vi "系列号查询.vi"() -> ()   [LabVIEW 2016, in "斯坦道多参数.lvlib"]
panel:
  in  "传感器系列号":T1
  in  "布尔":bool
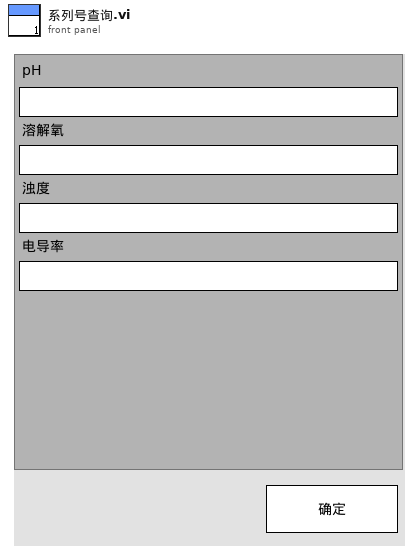
[diagram p1: front panel]
types:
  T1 = cluster{"pH":string, "溶解氧":string, "浊度":string, "电导率":string, "ORP":string, "叶绿素a":string, "藻密度":string}
  T2 = cluster{"pH探头选择":u16, "DO探头选择":u16, "电导率探头选择":u16, "浊度探头选择":u16, "叶绿素a探头选择":u16, "蓝绿藻探头选择":u16, "orp探头选择":u16, "COD探头选择":u16, "DO2探头选择":u16}
  T3 = cluster{"电极状态标志":u16, "电极型号标志":u16, "酸碱度测量值":sgl, "温度测量值":sgl, "酸碱度信号值":sgl, "温度信号值":sgl, "酸碱度偏移修正值":sgl, "温度偏移修正值":sgl, "手动温度补偿值":sgl, "酸碱度电极零点":sgl, "酸碱度电极斜率":sgl, "第1点标准值记录":sgl, "第1点信号值记录":sgl, "第1点温度值记录":sgl, "第2点标准值记录":sgl, "第2点信号值记录":sgl, "第2点温度值记录":sgl, "命令滤波设定":u16, "温度模式":enum16{"ATC", "MTC"}, "生产批次":u16, "电极序号":u16, "串口地址":u16, "串口波特率":enum16{"9600", "19200", "115200"}, "串口校验位":enum16{"NONE", "ODD", "EVEN"}, "串口停止位":enum16{"1bit", "2bit"}, "第一点标准值":sgl, "第二点标准值":sgl}
  T4 = cluster{"报警码":u16, "pH数值":sgl, "0X0003_NC":sgl, "温度数据":sgl, "pH原始信号 mv":sgl, "0X0009_NC":string, "产品名称":string, "序列号":string, "硬件版本":string, "软件版本":string, "通讯地址":u16, "波特率":u16, "设备类型":u16, "0X0026_NC":string, "第一点原始数据":sgl, "第一点校准数据":sgl, "第二点原始数据":sgl, "第二点校准数据":sgl, "探头校准命令":u16, "温度校准参数":sgl, "温度校准命令":u16}
  T5 = cluster{"电极状态标志":u16, "电极型号标志":u16, "溶解氧测量值":sgl, "温度测量值":sgl, "溶解氧饱和度值":sgl, "盐度补偿值":sgl, "大气压补偿值":sgl, "溶解氧偏移修正值":sgl, "温度偏移修正值":sgl, "手动温度补偿值":sgl, "溶解氧电极零点":sgl, "溶解氧电极斜率":sgl, "第1点标准值记录":sgl, "第1点信号值记录":sgl, "第1点温度值记录":sgl, "第2点标准值记录":sgl, "第2点信号值记录":sgl, "第2点温度值记录":sgl, "命令滤波设定":u16, "温度模式":enum16{"ATC", "MTC"}, "生产批次":u16, "电极序号":u16, "串口地址":u16, "串口波特率":enum16{"9600", "19200", "115200"}, "串口校验位":enum16{"NONE", "ODD", "EVEN"}, "串口停止位":enum16{"1bit", "2bit"}, "第一点标准值":sgl, "第二点标准值":sgl}
  T6 = cluster{"报警码":u16, "溶解氧数值（mg/L）":sgl, "溶解氧数据（%）":sgl, "温度数据":sgl, "溶解氧原始信号 nA":sgl, "大气压力":sgl, "盐度":sgl, "0X0009_NC":string, "产品名称":string, "序列号":string, "硬件版本":string, "软件版本":string, "通讯地址":u16, "波特率":u16, "设备类型":u16, "0X0026_NC":string, "第一点原始数据":sgl, "第一点校准数据":sgl, "第二点原始数据":sgl, "第二点校准数据":sgl, "探头校准命令":u16, "温度校准参数":sgl, "温度校准命令":u16}
  T7 = cluster{"电极状态标志":u16, "电极型号标志":u16, "浊度测量值":sgl, "温度测量值":sgl, "浊度信号值":sgl, "浊度偏移修正值":sgl, "温度偏移修正值":sgl, "手动温度补偿值":sgl, "浊度电极零点":sgl, "浊度电极斜率":sgl, "第1点标准值记录":sgl, "第1点信号值记录":sgl, "第1点温度值记录":sgl, "第2点标准值记录":sgl, "第2点信号值记录":sgl, "第2点温度值记录":sgl, "命令滤波设定":u16, "温度模式":enum16{"ATC", "MTC"}, "生产批次":u16, "电极序号":u16, "串口地址":u16, "串口波特率":enum16{"9600", "19200", "115200"}, "串口校验位":enum16{"NONE", "ODD", "EVEN"}, "串口停止位":enum16{"1bit", "2bit"}, "第一点标准值":sgl, "第二点标准值":sgl, "第三点标准值":sgl}
  T8 = cluster{"报警码":u16, "浊度数值 NTU":sgl, "温度数据":sgl, "原始光强数值":u16, "量程":u16, "平均次数":u16, "清扫模式":u16, "清扫次数":u16, "清扫间隔分钟":u16, "0X000B_NC":string, "产品名称":string, "序列号":string, "硬件版本":string, "软件版本":string, "通讯地址":u16, "波特率":u16, "设备类型":u16, "0X0026_NC":string, "校准量程":u16, "第一点原始光强":u16, "第一点校准数据":sgl, "第二点原始光强":u16, "第二点校准数据":sgl, "第三点原始光强":u16, "第三点校准数据":sgl, "探头校准命令":u16, "温度校准参数":sgl, "温度校准命令":u16}
  T9 = cluster{"电极状态标志":u16, "电极型号标志":u16, "电导率测量值":sgl, "温度测量值":sgl, "电导率信号值":sgl, "温度信号值":sgl, "温度补偿系数":sgl, "电导率偏移修正值":sgl, "温度偏移修正值":sgl, "手动温度补偿值":sgl, "电导率电极零点":sgl, "电导率电极斜率":sgl, "命令滤波设定":u16, "温度模式":enum16{"ATC", "MTC"}, "生产批次":u16, "电极序号":u16, "串口地址":u16, "串口波特率":enum16{"9600", "19200", "115200"}, "串口校验位":enum16{"NONE", "ODD", "EVEN"}, "串口停止位":enum16{"1bit", "2bit"}, "第一点标准值":sgl, "第二点标准值":sgl}
  T10 = cluster{"报警码":u16, "电导率数据（uS/cm）":sgl, "0x0003 NC":sgl, "温度数据":sgl, "电导率原始信号电阻":sgl, "当前量程":u16, "温度补偿系数":sgl, "0X0009_NC":string, "产品名称":string, "序列号":string, "硬件版本":string, "软件版本":string, "通讯地址":u16, "波特率":u16, "设备类型":u16, "0X0026_NC":string, "第一点原始数据":sgl, "第一点校准数据":sgl, "0X0035_NC":sgl, "0X0037_NC":sgl, "探头校准命令":u16, "温度校准参数":sgl, "温度校准命令":u16}
  T11 = cluster{"电极状态标志":u16, "电极型号标志":u16, "测量值":sgl, "温度测量值":sgl, "信号值":sgl, "温度信号值":sgl, "000AH_NC":sgl, "偏移修正值":sgl, "温度偏移修正值":sgl, "手动温度补偿值":sgl, "命令滤波设定":u16, "温度模式":enum16{"ATC", "MTC"}, "生产批次":u16, "传感器序号":u16, "串口地址":u16, "串口波特率":enum16{"9600", "19200", "115200"}, "串口校验位":enum16{"NONE", "ODD", "EVEN"}, "串口停止位":enum16{"1bit", "2bit"}}
  T12 = cluster{"报警码":u16, "叶绿素a":sgl, "温度数据":sgl, "原始光强数值":u16, "量程":u16, "平均次数":u16, "清扫模式":u16, "清扫次数":u16, "清扫间隔分钟":u16, "0X000B_NC":string, "产品名称":string, "序列号":string, "硬件版本":string, "软件版本":string, "通讯地址":u16, "波特率":u16, "设备类型":u16, "0X0026_NC":string, "校准量程":u16, "第一点原始光强":u16, "第一点校准数据":sgl, "第二点原始光强":u16, "第二点校准数据":sgl, "第三点原始光强":u16, "第三点校准数据":sgl, "探头校准命令":u16, "温度校准参数":sgl, "温度校准命令":u16}
  T13 = cluster{"报警码":u16, "蓝绿藻":sgl, "温度数据":sgl, "原始光强数值":u16, "量程":u16, "平均次数":u16, "清扫模式":u16, "清扫次数":u16, "清扫间隔分钟":u16, "0X000B_NC":string, "产品名称":string, "序列号":string, "硬件版本":string, "软件版本":string, "通讯地址":u16, "波特率":u16, "设备类型":u16, "0X0026_NC":string, "校准量程":u16, "第一点原始光强":u16, "第一点校准数据":sgl, "第二点原始光强":u16, "第二点校准数据":sgl, "第三点原始光强":u16, "第三点校准数据":sgl, "探头校准命令":u16, "温度校准参数":sgl, "温度校准命令":u16}
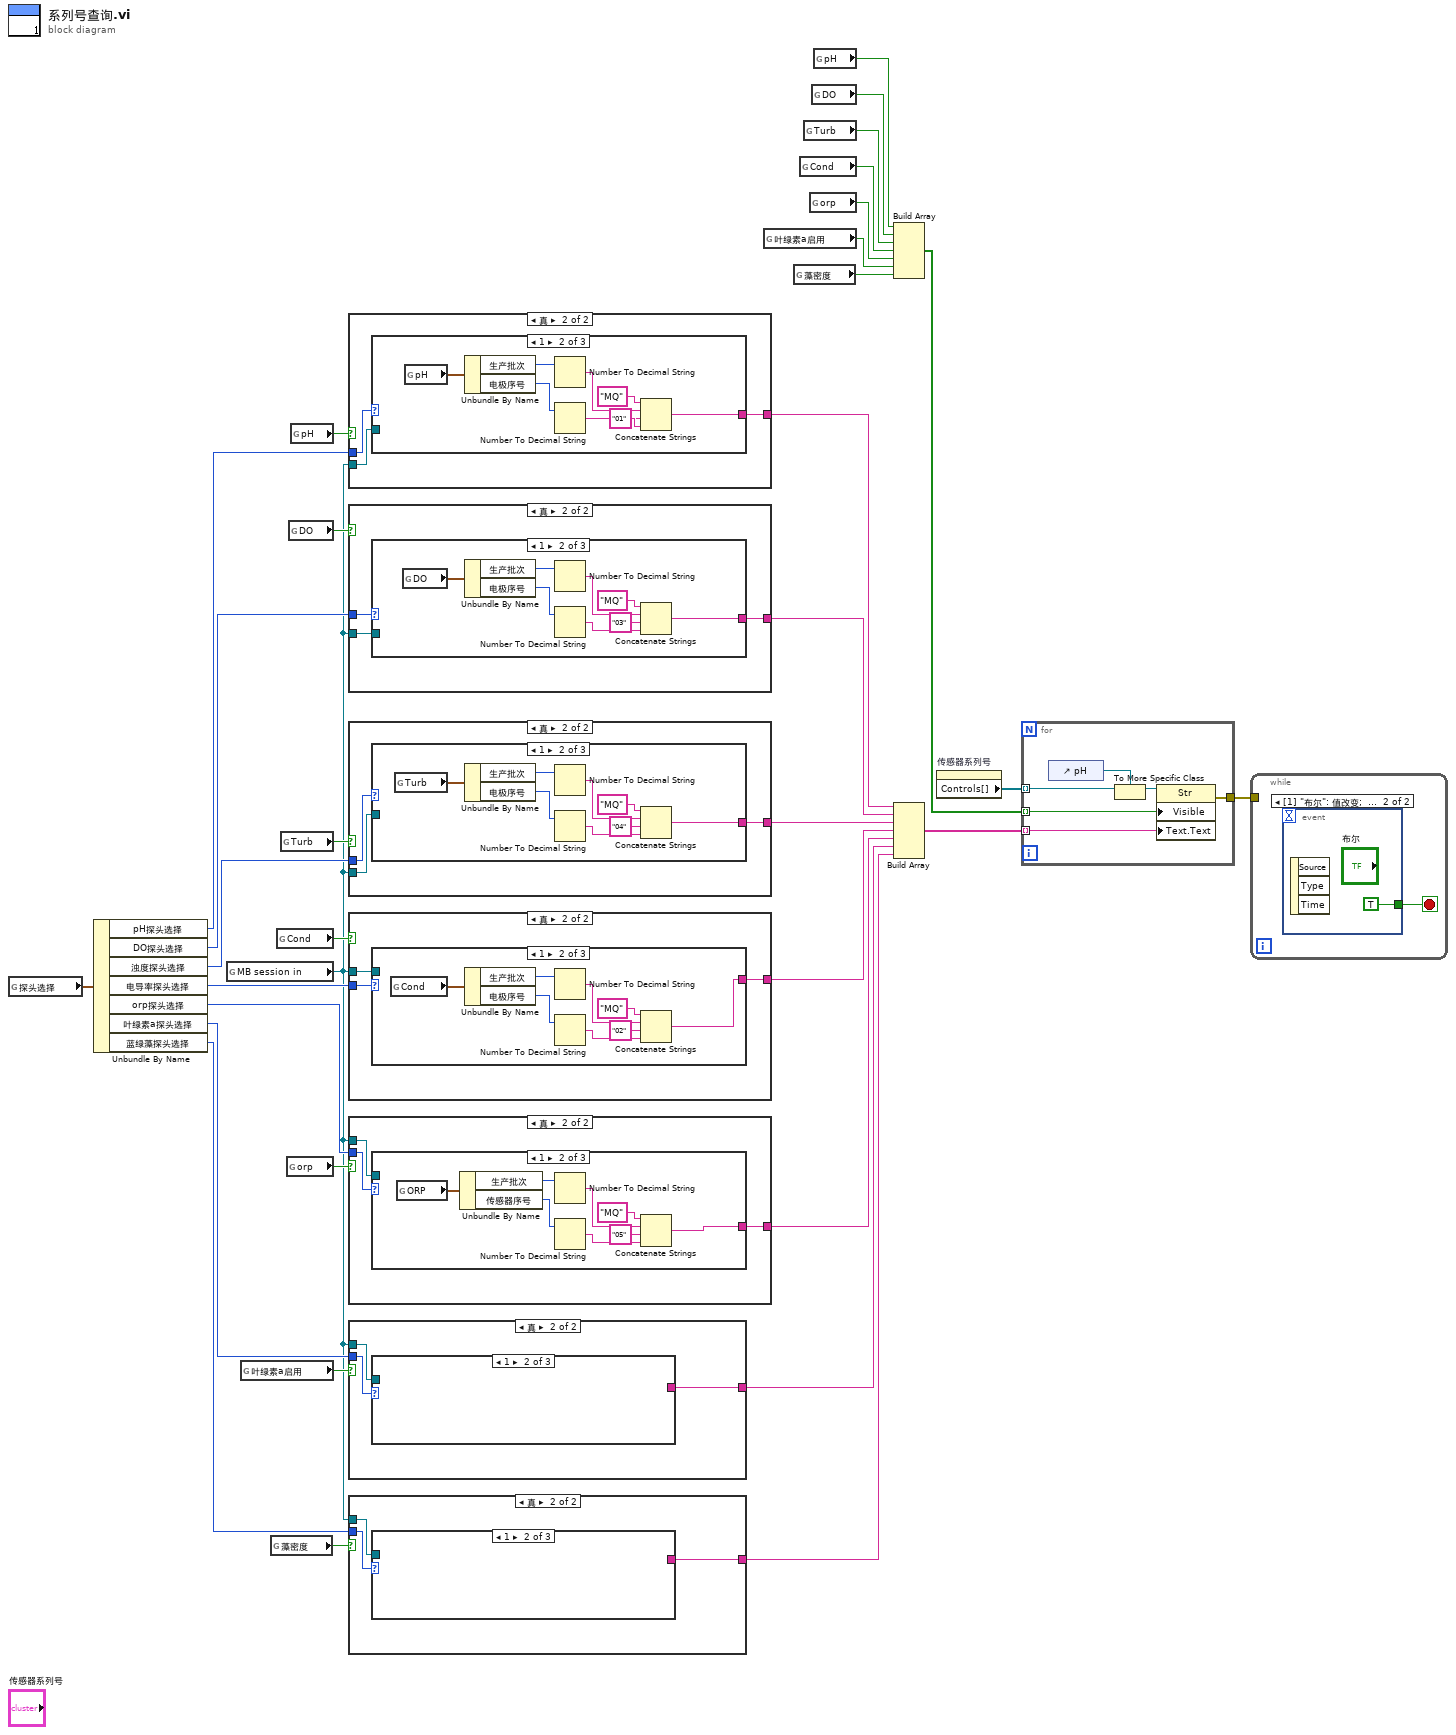
[diagram p0: block diagram]
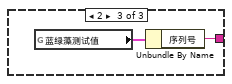
[diagram p4: hidden frame]
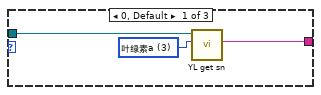
[diagram p6: hidden frame]
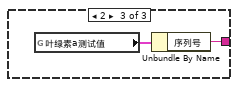
[diagram p7: hidden frame]
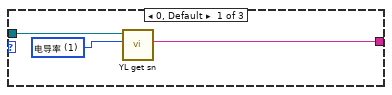
[diagram p12: hidden frame]
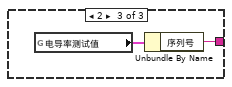
[diagram p13: hidden frame]
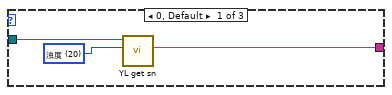
[diagram p15: hidden frame]
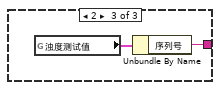
[diagram p16: hidden frame]
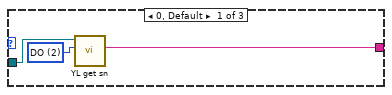
[diagram p18: hidden frame]
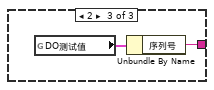
[diagram p19: hidden frame]
diagram:
  n1 = global read "断电保存变量.vi" "探头选择"() -> (w24:T2)
  n2 = Unbundle By Name(w24) -> ("pH探头选择"=w23:u16, "DO探头选择"=w21:u16, "浊度探头选择"=w19:u16, "电导率探头选择"=w16:u16, "orp探头选择"=w15:u16, "叶绿素a探头选择"=w13:u16, "蓝绿藻探头选择"=w9:u16)
  n3 = global read "多参数全局变量.vi" "MB session in"() -> (w10:refnum<class "MB_Master.lvclass">)
  n4 = global read "断电保存变量.vi" "叶绿素a启用"() -> (w12:bool)
  n5 = global read "断电保存变量.vi" "藻密度"() -> (w11:bool)
  n6 = global read "断电保存变量.vi" "Cond"() -> (w17:bool)
  n7 = global read "断电保存变量.vi" "Turb"() -> (w18:bool)
  n8 = global read "断电保存变量.vi" "orp"() -> (w14:bool)
  n9 = global read "断电保存变量.vi" "DO"() -> (w20:bool)
  n10 = global read "断电保存变量.vi" "pH"() -> (w22:bool)
  n11 = case shown="真" w22 {
    tunnel: w23 -> [_ w37]
    tunnel: [_ w36] -> w8
    tunnel: w10 -> [_ w35]
    frame False {
    }
    frame True {
      n12 = case shown="1" w37 {
        tunnel: w35 -> [w39 _ _]
        tunnel: [w38 w44 w49] -> w36
        frame 0, Default {
          w40 = u16 4 items=["电导率"=1, "DO"=2, "叶绿素a"=3, "pH"=4, "浊度"=20] ("探头型号")
          n13 = call "YL get sn.vi"("探头型号"=w40, "MB session in"=w39) -> ("SN"=w38:string)  [unwired: 7 in, 2 out]
        }
        frame 1 {
          n14 = global read "国弘过程全局变量.vi" "pH"() -> (w45:T3)
          n15 = Unbundle By Name(w45) -> ("生产批次"=w46:u16, "电极序号"=w47:u16)
          n16 = Number To Decimal String(number=w46) -> (decimal integer string=w48:string)  [unwired: 1 in]
          n17 = Number To Decimal String(number=w47) -> (decimal integer string=w42:string)  [unwired: 1 in]
          n18 = Concatenate Strings("MQ" ("字符串"), w48, "01" ("字符串"), w42) -> (w44:string)
        }
        frame 2 {
          n19 = global read "纳清过程全局变量.vi" "pH测试值"() -> (w50:T4)
          n20 = Unbundle By Name(w50) -> ("序列号"=w49:string)
        }
      }
    }
  }
  n21 = case shown="真" w20 {
    tunnel: w21 -> [_ w53]
    tunnel: [_ w52] -> w7
    tunnel: w10 -> [_ w51]
    frame False {
    }
    frame True {
      n22 = case shown="1" w53 {
        tunnel: w51 -> [w55 _ _]
        tunnel: [w54 w60 w65] -> w52
        frame 0, Default {
          w56 = u16 2 items=["电导率"=1, "DO"=2, "叶绿素a"=3, "pH"=4, "浊度"=20] ("探头型号")
          n23 = call "YL get sn.vi"("探头型号"=w56, "MB session in"=w55) -> ("SN"=w54:string)  [unwired: 7 in, 2 out]
        }
        frame 1 {
          n24 = global read "国弘过程全局变量.vi" "DO"() -> (w61:T5)
          n25 = Unbundle By Name(w61) -> ("生产批次"=w62:u16, "电极序号"=w63:u16)
          n26 = Number To Decimal String(number=w62) -> (decimal integer string=w64:string)  [unwired: 1 in]
          n27 = Number To Decimal String(number=w63) -> (decimal integer string=w58:string)  [unwired: 1 in]
          n28 = Concatenate Strings("MQ" ("字符串"), w64, "03" ("字符串"), w58) -> (w60:string)
        }
        frame 2 {
          n29 = global read "纳清过程全局变量.vi" "DO测试值"() -> (w66:T6)
          n30 = Unbundle By Name(w66) -> ("序列号"=w65:string)
        }
      }
    }
  }
  n31 = case shown="真" w18 {
    tunnel: w19 -> [_ w69]
    tunnel: [_ w68] -> w6
    tunnel: w10 -> [_ w67]
    frame False {
    }
    frame True {
      n32 = case shown="1" w69 {
        tunnel: w67 -> [w71 _ _]
        tunnel: [w70 w76 w81] -> w68
        frame 0, Default {
          w72 = u16 20 items=["电导率"=1, "DO"=2, "叶绿素a"=3, "pH"=4, "浊度"=20] ("探头型号")
          n33 = call "YL get sn.vi"("探头型号"=w72, "MB session in"=w71) -> ("SN"=w70:string)  [unwired: 7 in, 2 out]
        }
        frame 1 {
          n34 = global read "国弘过程全局变量.vi" "Turb"() -> (w77:T7)
          n35 = Unbundle By Name(w77) -> ("生产批次"=w78:u16, "电极序号"=w79:u16)
          n36 = Number To Decimal String(number=w78) -> (decimal integer string=w80:string)  [unwired: 1 in]
          n37 = Number To Decimal String(number=w79) -> (decimal integer string=w74:string)  [unwired: 1 in]
          n38 = Concatenate Strings("MQ" ("字符串"), w80, "04" ("字符串"), w74) -> (w76:string)
        }
        frame 2 {
          n39 = global read "纳清过程全局变量.vi" "浊度测试值"() -> (w82:T8)
          n40 = Unbundle By Name(w82) -> ("序列号"=w81:string)
        }
      }
    }
  }
  n41 = case shown="真" w17 {
    tunnel: w16 -> [_ w85]
    tunnel: [_ w84] -> w5
    tunnel: w10 -> [_ w83]
    frame False {
    }
    frame True {
      n42 = case shown="1" w85 {
        tunnel: w83 -> [w87 _ _]
        tunnel: [w86 w92 w97] -> w84
        frame 0, Default {
          w88 = u16 1 items=["电导率"=1, "DO"=2, "叶绿素a"=3, "pH"=4, "浊度"=20] ("探头型号")
          n43 = call "YL get sn.vi"("探头型号"=w88, "MB session in"=w87) -> ("SN"=w86:string)  [unwired: 7 in, 2 out]
        }
        frame 1 {
          n44 = global read "国弘过程全局变量.vi" "Cond"() -> (w93:T9)
          n45 = Unbundle By Name(w93) -> ("生产批次"=w94:u16, "电极序号"=w95:u16)
          n46 = Number To Decimal String(number=w94) -> (decimal integer string=w96:string)  [unwired: 1 in]
          n47 = Number To Decimal String(number=w95) -> (decimal integer string=w90:string)  [unwired: 1 in]
          n48 = Concatenate Strings("MQ" ("字符串"), w96, "02" ("字符串"), w90) -> (w92:string)
        }
        frame 2 {
          n49 = global read "纳清过程全局变量.vi" "电导率测试值"() -> (w98:T10)
          n50 = Unbundle By Name(w98) -> ("序列号"=w97:string)
        }
      }
    }
  }
  n51 = case shown="真" w14 {
    tunnel: w15 -> [_ w101]
    tunnel: [_ w100] -> w4
    tunnel: w10 -> [_ w99]
    frame False {
    }
    frame True {
      n52 = case shown="1" w101 {
        tunnel: w99 -> [_ _ _]
        tunnel: [_ w105 _] -> w100
        frame 0, Default {
        }
        frame 1 {
          n53 = global read "国弘过程全局变量.vi" "ORP"() -> (w106:T11)
          n54 = Unbundle By Name(w106) -> ("生产批次"=w107:u16, "传感器序号"=w108:u16)
          n55 = Number To Decimal String(number=w107) -> (decimal integer string=w109:string)  [unwired: 1 in]
          n56 = Number To Decimal String(number=w108) -> (decimal integer string=w103:string)  [unwired: 1 in]
          n57 = Concatenate Strings("MQ" ("字符串"), w109, "05" ("字符串"), w103) -> (w105:string)
        }
        frame 2 {
        }
      }
    }
  }
  n58 = case shown="真" w12 {
    tunnel: w13 -> [_ w112]
    tunnel: [_ w111] -> w3
    tunnel: w10 -> [_ w110]
    frame False {
    }
    frame True {
      n59 = case shown="1" w112 {
        tunnel: w110 -> [w114 _ _]
        tunnel: [w113 _ w116] -> w111
        frame 0, Default {
          w115 = u16 3 items=["电导率"=1, "DO"=2, "叶绿素a"=3, "pH"=4, "浊度"=20] ("探头型号")
          n60 = call "YL get sn.vi"("探头型号"=w115, "MB session in"=w114) -> ("SN"=w113:string)  [unwired: 7 in, 2 out]
        }
        frame 1 {
        }
        frame 2 {
          n61 = global read "纳清过程全局变量.vi" "叶绿素a测试值"() -> (w117:T12)
          n62 = Unbundle By Name(w117) -> ("序列号"=w116:string)
        }
      }
    }
  }
  n63 = case shown="真" w11 {
    tunnel: w9 -> [_ w120]
    tunnel: [_ w119] -> w2
    tunnel: w10 -> [_ w118]
    frame False {
    }
    frame True {
      n64 = case shown="1" w120 {
        tunnel: w118 -> [_ _ _]
        tunnel: [_ _ w121] -> w119
        frame 0, Default {
        }
        frame 1 {
        }
        frame 2 {
          n65 = global read "纳清过程全局变量.vi" "蓝绿藻测试值"() -> (w122:T13)
          n66 = Unbundle By Name(w122) -> ("序列号"=w121:string)
        }
      }
    }
  }
  n67 = global read "断电保存变量.vi" "叶绿素a启用"() -> (w29:bool)
  n68 = global read "断电保存变量.vi" "藻密度"() -> (w28:bool)
  n69 = global read "断电保存变量.vi" "Cond"() -> (w31:bool)
  n70 = global read "断电保存变量.vi" "Turb"() -> (w32:bool)
  n71 = global read "断电保存变量.vi" "orp"() -> (w30:bool)
  n72 = global read "断电保存变量.vi" "DO"() -> (w33:bool)
  n73 = global read "断电保存变量.vi" "pH"() -> (w34:bool)
  n74 = Build Array(w34, w33, w32, w31, w30, w29, w28) -> (w26:bool[])
  n75 = Build Array(w8, w7, w6, w5, w4, w3, w2) -> (w1:string[])
  n76 = property on="传感器系列号" class="Clust (严格)"() -> ("Controls[]"=w27:refnum<vi>[])  [unwired: 2 in, 2 out]
  n77 = for {
    tunnel: w27 -> [w126] mode=indexing
    tunnel: w26 -> [w128] mode=indexing
    tunnel: [w127] -> w25
    tunnel: w1 -> [w123] mode=indexing
    n78 = control-ref of="pH"() -> (w125:refnum<vi>)
    n79 = To More Specific Class(target class=w125, reference=w126) -> (specific class reference=w124:refnum<vi>)  [unwired: 1 in, 1 out]
    n80 = property class="Str"(reference=w124, "Visible"=w128, "Text.Text"=w123) -> (error out=w127:errorcluster)  [unwired: 1 in, 1 out]
  }
  n81 = while {
    tunnel: w25 -> [_]
    stop <- w129 stop-if-true
    n82 = event shown="[1] \"布尔\": 值改变;  前面板关闭" {
      selector: _ -> [_ _]
      dyn-events: _ -> [_ _]
      timeout: _ -> [_ _]
      tunnel: [_ TRUE] -> w129
      event Timeout {
        n83 = event-data() -> ()  [unwired: 1 in, 3 out]
      }
      event "布尔": Value Change; Panel Close {
        n84 = event-data() -> ()  [unwired: 1 in, 3 out]
      }
    }
  }
